vi "Pre-Process.vi"(11 "Laser in":refnum<class "Laser.lvclass">) -> (3 "Laser out":refnum<class "Laser.lvclass">)   [LabVIEW 2021, in "Laser.lvclass"]
uses:
  Laser.lvclass
  Element/Element.lvclass
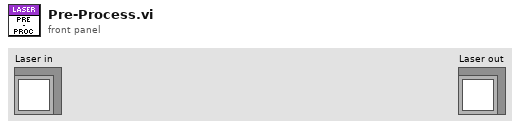
[diagram p1: front panel]
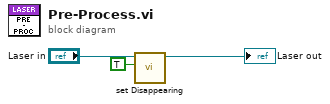
[diagram p0: block diagram]
diagram:
  n1 = call "set Disappearing.vi"("Disappearing"=TRUE, "Element in"="Laser in") -> ("Element out"=→"Laser out":refnum<class "Laser.lvclass">)  [unwired: 9 in]
